vi "Save Data.vi"(0 "Experiment Indicator":string, 1 "Username":string, 5 "Pixel":dbl, 7 "Scan direction":i32, 9 "Data Array":dbl[][](array[numeric]), 11 "Cell details cluster":T1={"Measure?"=TRUE, "Area (cm^2)"=0.0, "Cell Label"="", "Cell Description"="", "Cell Position"=0, "Time in rig (s)"=0.0, "Time to next scan (s)"=0.0, "Scan number"=0.0, "When did you stick it in?"=0.0, "Time between scans (s)"=0.0, "Time of the last scan (s)"=0.0, "Scan settings in queue"=0, "Sample Holder"=0.0} {"Scan settings in queue" items=["Regular", "Inverted"]; "Time of the last scan (s)" format="%<%H:%M:%S>t"; "When did you stick it in?" format="%<%H:%M:%S>t"; "Time to next scan (s)" format="%<%H:%M:%S>t"; "Time in rig (s)" format="%<%H:%M:%S>t"}, 12 "Show me Scan \nSettings JV set":T2={"Light Intensity (Suns)"=1.0, "Stabilization Time (s)"=5.0, "Maximum Voltage (V)"=0.0, "Minimum Voltage (V)"=-1.0, "Range Options"=0, "Scan Direction\nDU (T), UD (F)"=TRUE, "Step Size (V)"=0.01, "Source Delay (s)"=0.15} {"Range Options" items=["Auto Range", "Semi-Auto Range", "100 uA", "1 mA", "10 mA", "100 mA", "1A"]}, 13 "Time zero":timestamp) -> (4 "Master Log":string[][](table), 6 "File path for master log":path, 10 "File path for device log":path, 14 "File path for JV data":path, 15 "File path for JV image":path)   [LabVIEW 2011]
uses:
  <vilib>/Utility/file.llb/Write To Spreadsheet File (string).vi
  <vilib>/Utility/file.llb/Read From Spreadsheet File (string).vi
  <vilib>/Analysis/NI_AALPro.lvlib
panel:
  out "PCE":dbl
  out "FF":dbl
  out "Voc":dbl
  out "Jsc":dbl
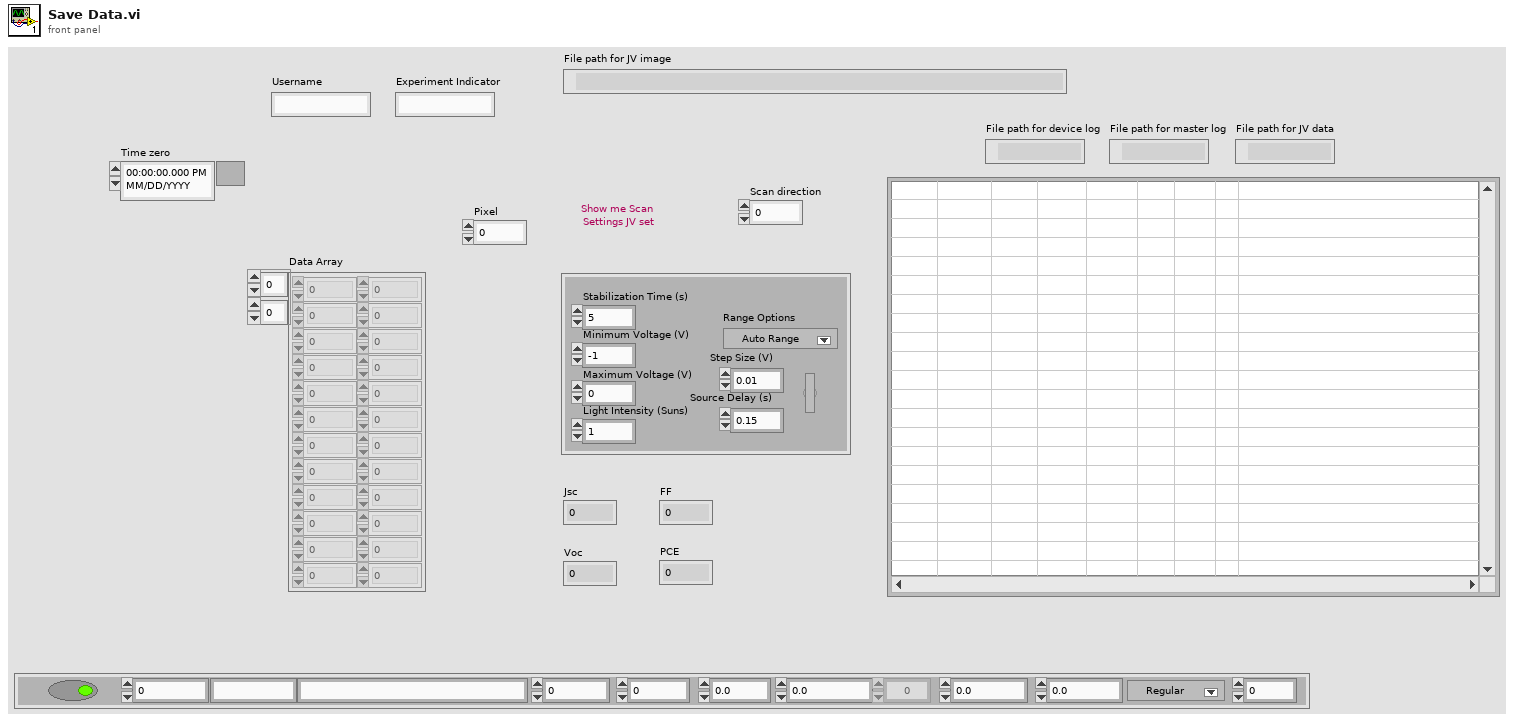
[diagram p1: front panel]
types:
  T1 = cluster{"Measure?":bool, "Area (cm^2)":dbl, "Cell Label":string, "Cell Description":string, "Cell Position":i32, "Time in rig (s)":dbl, "Time to next scan (s)":dbl, "Scan number":dbl, "When did you stick it in?":dbl, "Time between scans (s)":dbl, "Time of the last scan (s)":dbl, "Scan settings in queue":u16, "Sample Holder":dbl}
  T2 = cluster{"Light Intensity (Suns)":dbl, "Stabilization Time (s)":dbl, "Maximum Voltage (V)":dbl, "Minimum Voltage (V)":dbl, "Range Options":u16, "Scan Direction\nDU (T), UD (F)":bool, "Step Size (V)":dbl, "Source Delay (s)":dbl}
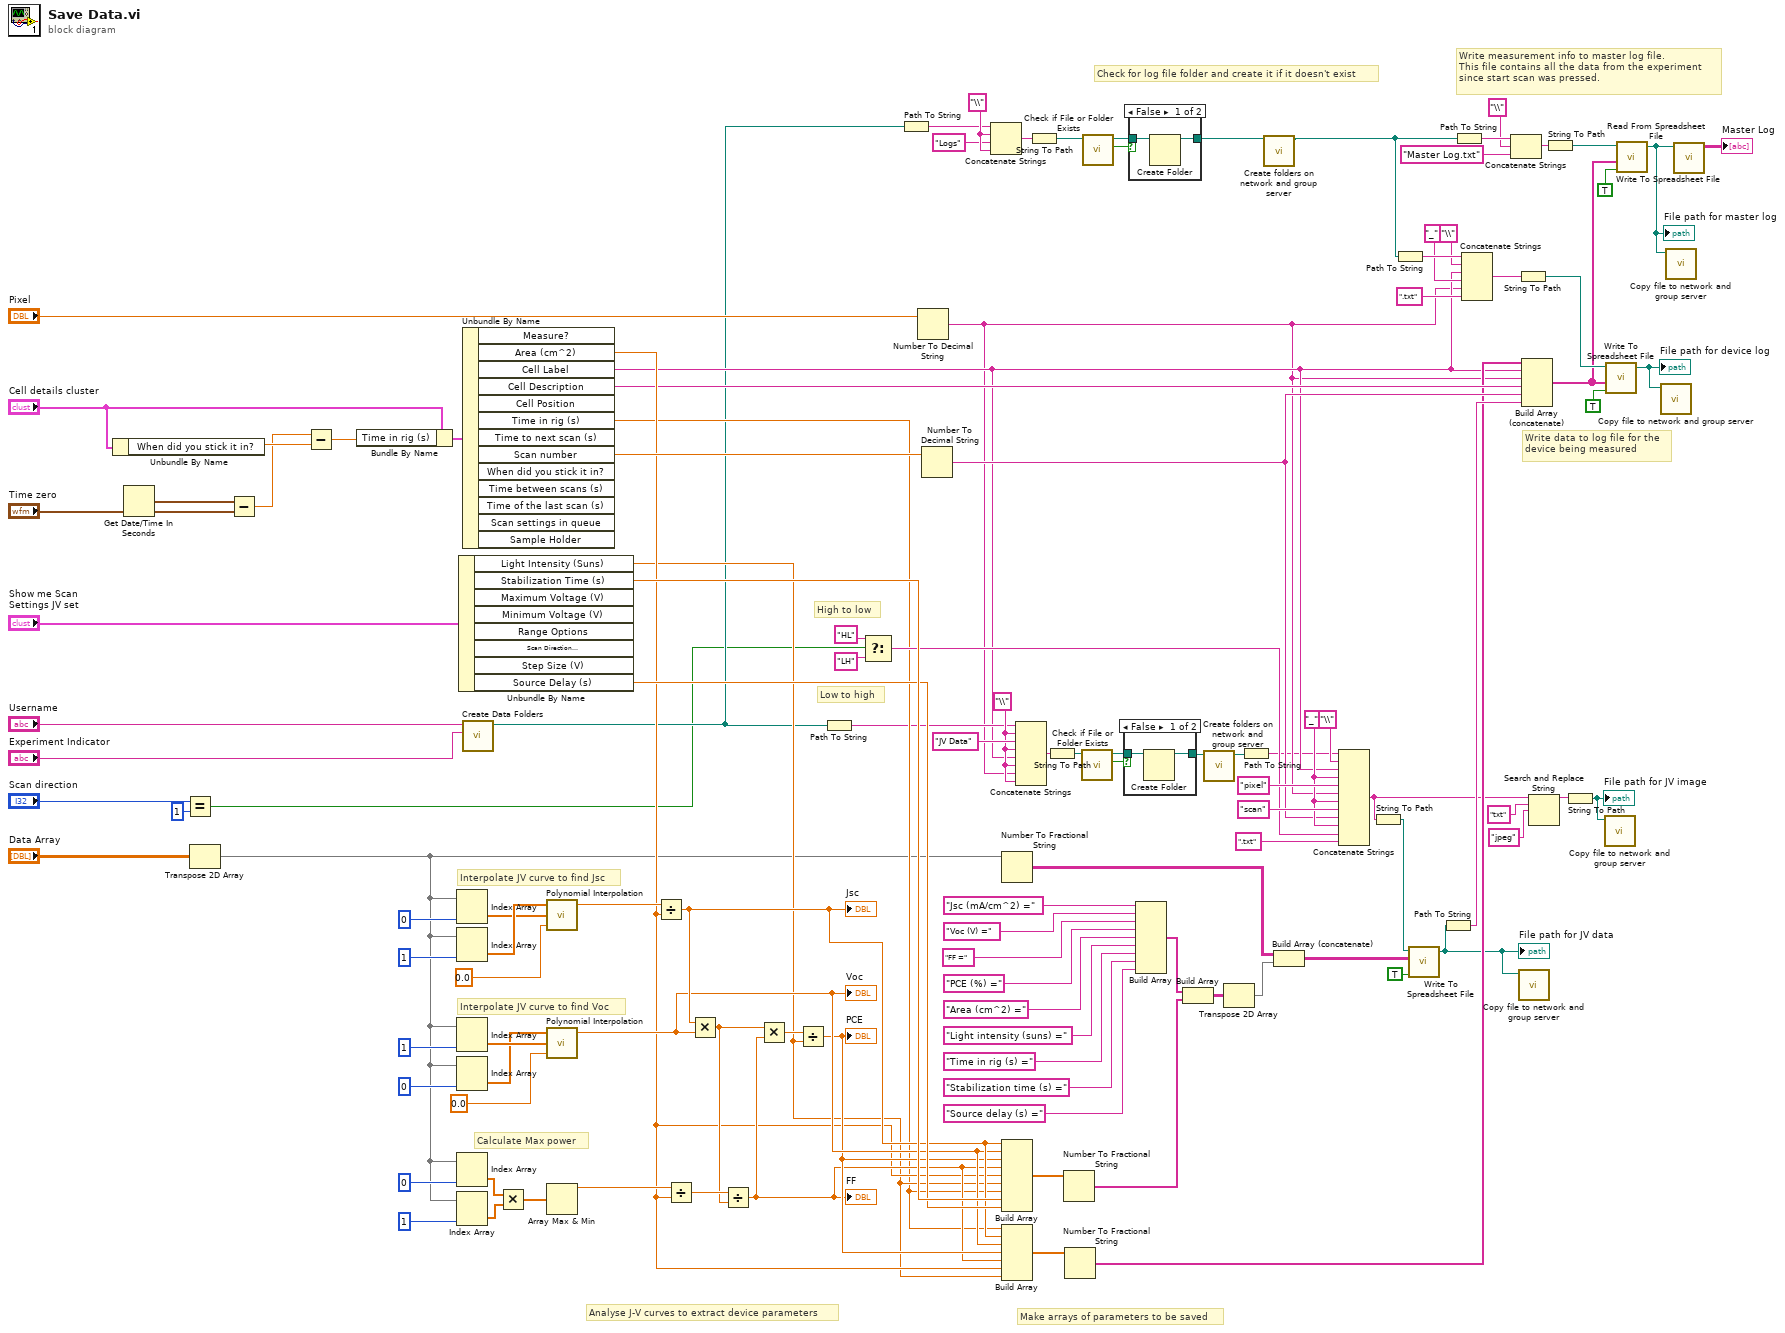
[diagram p0: block diagram]
diagram:
  w34 = "\\"
  w60 = "\\"
  w78 = "_"
  # "Make arrays of parameters to be saved"
  # "Calculate Max power"
  # "Interpolate JV curve to find Voc"
  # "Interpolate JV curve to find Jsc"
  # "Analyse J-V curves to extract device parameters"
  # "Write data to log file for the\ndevice being measured"
  # "Write measurement info to master log file.\nThis file contains all the data from the experiment\nsince start scan was pressed."
  # "Check for log file folder and create it if it doesn't exist"
  # "Low to high"
  # "High to low"
  n1 = Unbundle By Name("Cell details cluster") -> ("When did you stick it in?"=w18:dbl)
  n2 = Get Date/Time In Seconds() -> (seconds since 1Jan1904=w19:timestamp)
  n3 = Equal?(x="Scan direction", y=1) -> (x = y?=w7:bool)
  n4 = Transpose 2D Array(2D array="Data Array") -> (transposed array=w11:dbl[][])
  n5 = Subtract(x=w19, y="Time zero") -> (x-y=w17:dbl)
  n6 = Subtract(x=w17, y=w18) -> (x-y=w15:dbl)
  n7 = Bundle By Name(cluster="Cell details cluster", "Time in rig (s)"=w15) -> (w20:T1)
  n8 = Index Array(array=w11, index (col)=0) -> (element=w108:dbl[])  [unwired: 1 in]
  n9 = Index Array(array=w11, index (col)=1) -> (element=w109:dbl[])  [unwired: 1 in]
  n10 = Index Array(array=w11, index (col)=1) -> (element=w107:dbl[])  [unwired: 1 in]
  n11 = Index Array(array=w11, index (col)=0) -> (element=w104:dbl[])  [unwired: 1 in]
  n12 = Index Array(array=w11, index (col)=0) -> (element=w115:dbl[])  [unwired: 1 in]
  n13 = Index Array(array=w11, index (col)=1) -> (element=w114:dbl[])  [unwired: 1 in]
  n14 = Unbundle By Name("Show me Scan \nSettings JV set") -> ("Light Intensity (Suns)"=w68:dbl, "Stabilization Time (s)"=w88:dbl, "Source Delay (s)"=w87:dbl)  [unwired: 5 out]
  n15 = Unbundle By Name(w20) -> ("Area (cm^2)"=w69:dbl, "Cell Label"=w32:string, "Cell Description"=w66:string, "Time in rig (s)"=w67:dbl, "Scan number"=w83:dbl)  [unwired: 8 out]
  n16 = call "Create Data Folders.vi"("Experiment Indicator"="Experiment Indicator", "username"="Username") -> ("Data Output Folder"=w26:path)  [unwired: 9 in]
  n17 = Multiply(x=w115, y=w114) -> (x*y=w105:dbl[])
  n18 = call <vilib>:"Polynomial Interpolation.vi"("x value"=0.0, "X"=w108, "Y"=w109) -> ("interpolation value"=w112:dbl)  [unwired: 2 out]
  n19 = call <vilib>:"Polynomial Interpolation.vi"("x value"=0.0, "X"=w107, "Y"=w104) -> ("interpolation value"=w72:dbl)  [unwired: 2 out]
  "Voc" <- w72
  n20 = Array Max & Min(array=w105) -> (max value=w106:dbl)  [unwired: 3 out]
  n21 = Divide(x=w112, y=w69) -> (x/y=w73:dbl)
  "Jsc" <- w73
  n22 = Divide(x=w106, y=w69) -> (x/y=w103:dbl)
  n23 = Multiply(x=w73, y=w72) -> (x*y=w102:dbl)
  n24 = Divide(x=w103, y=w102) -> (x/y=w70:dbl)
  "FF" <- w70
  n25 = Multiply(x=w102, y=w70) -> (x*y=w113:dbl)
  n26 = Divide(x=w113, y=w68) -> (x/y=w71:dbl)
  "PCE" <- w71
  n27 = Path To String(path=w26) -> (string=w33:string)
  n28 = Select(t="HL", s=w7, f="LH") -> (s? t:f=w77:string)
  n29 = Path To String(path=w26) -> (string=w57:string)
  n30 = Number To Decimal String(number="Pixel") -> (decimal integer string=w31:string)  [unwired: 1 in]
  n31 = Number To Decimal String(number=w83) -> (decimal integer string=w65:string)  [unwired: 1 in]
  n32 = Concatenate Strings(w57, w60, "Logs", w60) -> (w58:string)
  n33 = Number To Fractional String(number=w11) -> (F-format string=w10:string[][])  [unwired: 3 in]
  n34 = Build Array(w73, w72, w71, w70, w69, w68, w67, w88, w87) -> (w97:dbl[])
  n35 = Build Array(w67, w73, w72, w71, w70, w69, w68) -> (w63:dbl[])
  n36 = Concatenate Strings(w33, w34, "JV Data", w34, w32, w34, w31, w34) -> (w38:string)
  n37 = String To Path(string=w58) -> (path=w56:path)
  n38 = String To Path(string=w38) -> (path=w37:path)
  n39 = Number To Fractional String(number=w97) -> (F-format string=w95:string[])  [unwired: 3 in]
  n40 = Number To Fractional String(number=w63) -> (F-format string=w62:string[])  [unwired: 3 in]
  n41 = call <vilib>:"Check if File or Folder Exists.vi"("path"=w37) -> ("file or folder exists?"=w36:bool, "dup path"=w35:path)  [unwired: 8 in, 1 out]
  n42 = call <vilib>:"Check if File or Folder Exists.vi"("path"=w56) -> ("file or folder exists?"=w55:bool, "dup path"=w54:path)  [unwired: 8 in, 1 out]
  n43 = case shown="False" w36 {
    tunnel: w35 -> [w124 w125]
    tunnel: [w123 w125] -> w3
    frame False {
      n44 = Create Folder(path (use dialog)=w124) -> (created path=w123:path)  [unwired: 2 in, 2 out]
    }
    frame True {
    }
  }
  n45 = case shown="False" w55 {
    tunnel: w54 -> [w127 w128]
    tunnel: [w126 w128] -> w5
    frame False {
      n46 = Create Folder(path (use dialog)=w127) -> (created path=w126:path)  [unwired: 2 in, 2 out]
    }
    frame True {
    }
  }
  n47 = Build Array("Jsc (mA/cm^2) =", "Voc (V) =", "FF =", "PCE (%) =", "Area (cm^2) =", "Light intensity (suns) =", "Time in rig (s) =", "Stabilization time (s) =", "Source delay (s) =") -> (w96:string[])
  n48 = Build Array(w96, w95) -> (w86:string[][])
  n49 = call "Create folders on network and group server.vi"("File path in"=w3) -> ("File path out"=w2:path)  [unwired: 10 in]
  n50 = Transpose 2D Array(2D array=w86) -> (transposed array=w85:string[][])
  n51 = Path To String(path=w2) -> (string=w30:string)
  n52 = call "Create folders on network and group server.vi"("File path in"=w5) -> ("File path out"=w4:path)  [unwired: 10 in]
  n53 = Build Array (concatenate)(w10, w85) -> (w94:string[][])
  n54 = Concatenate Strings(w30, "\\", w32, w78, "pixel", w31, w78, "scan", w65, w78, w77, ".txt") -> (w29:string)
  n55 = String To Path(string=w29) -> (path=w75:path)
  n56 = Path To String(path=w4) -> (string=w53:string)
  n57 = call-poly <vilib>:"Write To Spreadsheet File.vi"("append to file? (new file:F)"=TRUE, "2D data"=w94, "file path (dialog if empty)"=w75) -> ("new file path (Not A Path if cancelled)"=w1:path)  [unwired: 5 in]
  "File path for JV data" <- w1
  n58 = Path To String(path=w1) -> (string=w64:string)
  n59 = Path To String(path=w4) -> (string=w49:string)
  n60 = Concatenate Strings(w53, "\\", w32, "_", w31, ".txt") -> (w51:string)
  n61 = Concatenate Strings(w49, "\\", "Master Log.txt") -> (w46:string)
  n62 = String To Path(string=w51) -> (path=w50:path)
  n63 = call "Copy file to network and group server.vi"("File path in"=w1) -> ()  [unwired: 11 in]
  n64 = Build Array (concatenate)(w62, w32, w31, w66, w65, w64) -> (w44:string[])
  n65 = Search and Replace String(input string=w29, search string="txt", replace string="jpeg") -> (result string=w28:string)  [unwired: 5 in, 3 out]
  n66 = String To Path(string=w46) -> (path=w45:path)
  n67 = String To Path(string=w28) -> (path=w23:path)
  "File path for JV image" <- w23
  n68 = call "Copy file to network and group server.vi"("File path in"=w23) -> ()  [unwired: 11 in]
  n69 = call-poly <vilib>:"Write To Spreadsheet File.vi"("append to file? (new file:F)"=TRUE, "1D data"=w44, "file path (dialog if empty)"=w50) -> ("new file path (Not A Path if cancelled)"=w22:path)  [unwired: 5 in]
  "File path for device log" <- w22
  n70 = call-poly <vilib>:"Write To Spreadsheet File.vi"("append to file? (new file:F)"=TRUE, "1D data"=w44, "file path (dialog if empty)"=w45) -> ("new file path (Not A Path if cancelled)"=w21:path)  [unwired: 5 in]
  "File path for master log" <- w21
  n71 = call "Copy file to network and group server.vi"("File path in"=w22) -> ()  [unwired: 11 in]
  n72 = call "Copy file to network and group server.vi"("File path in"=w21) -> ()  [unwired: 11 in]
  n73 = call-poly <vilib>:"Read From Spreadsheet File.vi"("file path (dialog if empty)"=w21) -> ("all rows"=→"Master Log":string[][])  [unwired: 6 in, 4 out]
